vi "Test shm accept Command set Log Level LV.vi"(8 "error in (no error)":errorcluster, 11 "command_setLogLevel_Ctl":cluster{"level":i32}) -> (0 "error out":errorcluster, 2 "function return":i32, 3 "command_setLogLevel_Ctl out":cluster{"level":i32})   [LabVIEW 2018, in "SALLV_Test.lvlib"]
doc: "int Test_shm_acceptCommand_setLogLevelLV(Test_command_setLogLevelLV *command_setLogLevel_Ctl );"
uses:
  SALLV_Test.lvlib
  SALLV_Test.so
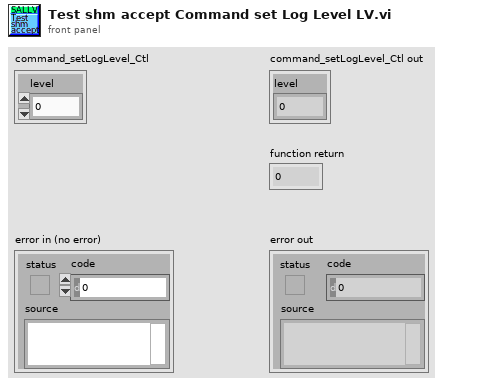
[diagram p1: front panel]
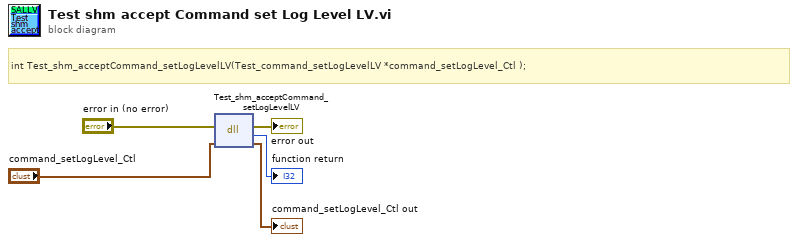
[diagram p0: block diagram]
diagram:
  # "int Test_shm_acceptCommand_setLogLevelLV(Test_command_setLogLevelLV *command_setLogLevel_Ctl );"
  n1 = dll-call lib="home/ttsai/Documents/salLabVIEWtestData/SALLV_Test.*" fn="Test_shm_acceptCommand_setLogLevelLV"(error in="error in (no error)", "command_setLogLevel_Ctl"="command_setLogLevel_Ctl") -> (error out=→"error out":errorcluster, →"function return":i32, "command_setLogLevel_Ctl"=→"command_setLogLevel_Ctl out":cluster{"level":i32})  [unwired: 2 in, 1 out]
